vi "Pick Banana.vi"(5 "Strategies.Test":T1, 7 "Strategies.Assert":T2, 8 "error in":errorcluster, 9 "Ephemeral Strategies":map{string, refnum<class "BananaPeel.lvclass">}(c390), 10 "Peels":refnum<class "BananaPeel.lvclass">[](array[class]), 11 "Banana":refnum<class "Banana.lvclass">) -> (0 "error out":errorcluster, 3 "Banana":refnum<class "Banana.lvclass">)   [LabVIEW 2021, in "Bananas.lvlib"]
uses:
  Bananas.lvlib
  Banana/Banana.lvclass
  BananaPeel/BananaPeel.lvclass
  <vilib>/LabVIEW Open Source Project/Data Manipulation/Variant/OpenVariant.lvlib
  Platano/Platano.lvclass
  AssertTrue/AssertTrue.lvclass
  C:/Repositories/LVOS/Bananas/lv-src/Bananas/AssertTrue/AssertTrue.lvclass
  C:/Repositories/LVOS/Bananas/lv-src/Bananas/BananaPeel/BananaPeel.lvclass
  AssertFalse/AssertFalse.lvclass
  C:/Repositories/LVOS/Bananas/lv-src/Bananas/AssertFalse/AssertFalse.lvclass
  AssertEqualValue/AssertEqualValue.lvclass
  C:/Repositories/LVOS/Bananas/lv-src/Bananas/AssertEqualValue/AssertEqualValue.lvclass
  AssertEqualType/AssertEqualType.lvclass
  C:/Repositories/LVOS/Bananas/lv-src/Bananas/AssertEqualType/AssertEqualType.lvclass
  AssertCompareValue/AssertCompareValue.lvclass
  C:/Repositories/LVOS/Bananas/lv-src/Bananas/AssertCompareValue/AssertCompareValue.lvclass
  AssetError/AssertError.lvclass
  C:/Repositories/LVOS/Bananas/lv-src/Bananas/AssetError/AssertError.lvclass
  AssertAlmostEqual/AssertAlmostEqualValue.lvclass
  C:/Repositories/LVOS/Bananas/lv-src/Bananas/AssertAlmostEqual/AssertAlmostEqualValue.lvclass
  DefineTest/DefineTest.lvclass
  C:/Repositories/LVOS/Bananas/lv-src/Bananas/DefineTest/DefineTest.lvclass
  DefineSuite/DefineSuite.lvclass
  C:/Repositories/LVOS/Bananas/lv-src/Bananas/DefineSuite/DefineSuite.lvclass
  Assertion Strategies -- cluster.ctl
  Test Strategies -- cluster.ctl
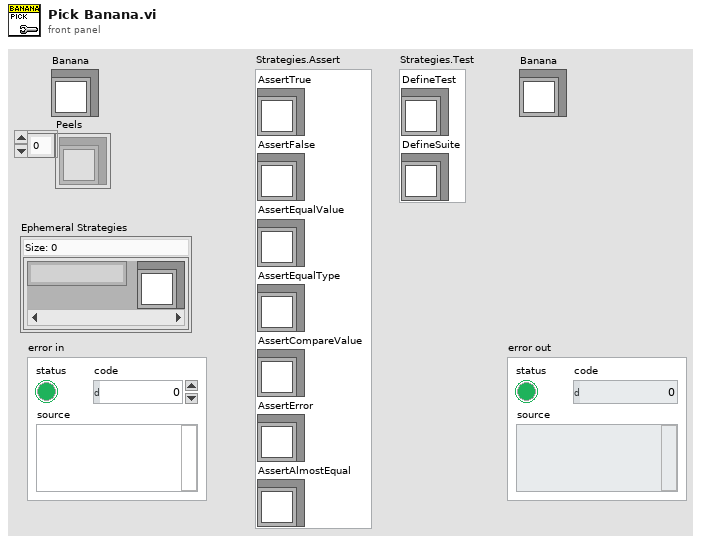
[diagram p1: front panel]
types:
  T1 = typedef "Bananas.lvlib/Test Strategies -- cluster.ctl" = cluster{"DefineTest":refnum<class "DefineTest.lvclass">, "DefineSuite":refnum<class "DefineSuite.lvclass">}
  T2 = typedef "Bananas.lvlib/Assertion Strategies -- cluster.ctl" = cluster{"AssertTrue":refnum<class "AssertTrue.lvclass">, "AssertFalse":refnum<class "AssertFalse.lvclass">, "AssertEqualValue":refnum<class "AssertEqualValue.lvclass">, "AssertEqualType":refnum<class "AssertEqualType.lvclass">, "AssertCompareValue":refnum<class "AssertCompareValue.lvclass">, "AssertError":refnum<class "AssertError.lvclass">, "AssertAlmostEqual":refnum<class "AssertAlmostEqualValue.lvclass">}
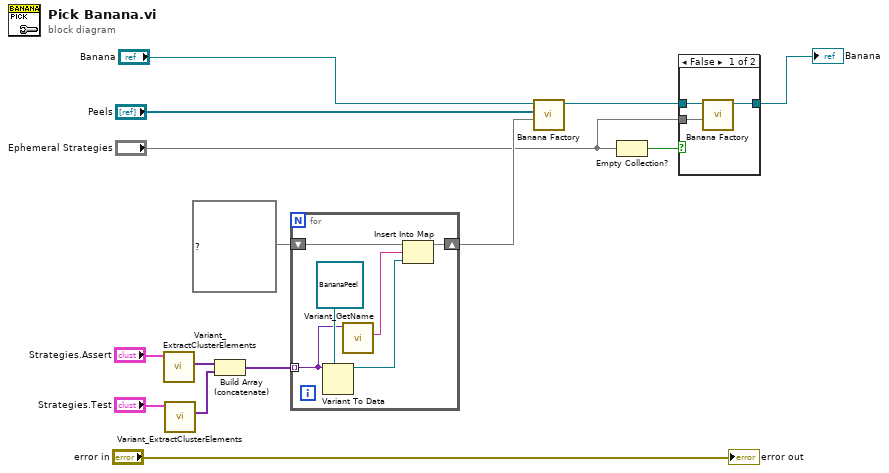
[diagram p0: block diagram]
diagram:
  n1 = call <vilib>:"Variant_ExtractClusterElements.vi"("Cluster"="Strategies.Assert") -> ("Elements"=w11:variant[])  [unwired: 8 in, 2 out]
  n2 = call <vilib>:"Variant_ExtractClusterElements.vi"("Cluster"="Strategies.Test") -> ("Elements"=w12:variant[])  [unwired: 8 in, 2 out]
  n3 = Build Array (concatenate)(w11, w12) -> (w10:variant[])
  n4 = for {
    tunnel: w10 -> [w19] mode=indexing
    shift-right: [w18] -> w7
    shift-left: map{string, refnum<class "BananaPeel.lvclass">} {} ("Ephemeral Strategies") -> [w17]
    n5 = Variant To Data(type=refnum<class "BananaPeel.lvclass"> refnum ("BananaPeel"), Variant=w19) -> (data=w15:refnum<class "BananaPeel.lvclass">)  [unwired: 1 in, 1 out]
    n6 = call <vilib>:"Variant_GetName.vi"("Variant"=w19) -> ("Name"=w16:string)  [unwired: 8 in, 2 out]
    n7 = Insert Into Map(map in=w17, key=w16, value=w15) -> (map out=w18:map{string, refnum<class "BananaPeel.lvclass">})  [unwired: 2 out]
  }
  n8 = call "Banana Factory.vi"("Strategies"=w7, "Peels"="Peels", "Platano"="Banana") -> ("Banana"=w5:refnum<class "Banana.lvclass">)  [unwired: 8 in]
  n9 = Empty Collection?(1:"Ephemeral Strategies") -> (0:w2:bool)
  n10 = case shown="False" w2 {
    tunnel: "Ephemeral Strategies" -> [w23 _]
    tunnel: w5 -> [w22 w24]
    tunnel: [w21 w24] -> w4
    frame False {
      n11 = call "Banana Factory.vi"("Strategies"=w23, "Platano"=w22) -> ("Banana"=w21:refnum<class "Banana.lvclass">)  [unwired: 9 in]
    }
    frame True {
    }
  }
  "Banana" <- w4
  "error out" <- "error in"
